vi "Wavechart erstellen.vi"(1 "file path (dialog if empty)":path) -> (0 "XY Graph":cluster{timestamp[], dbl[]}[](graph))   [LabVIEW 2021]
uses:
  <vilib>/Utility/file.llb/Read Delimited Spreadsheet (string).vi
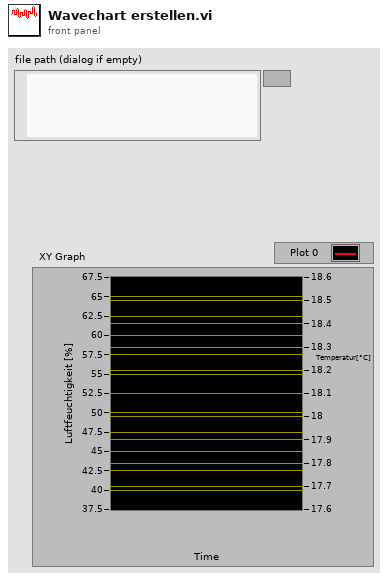
[diagram p1: front panel]
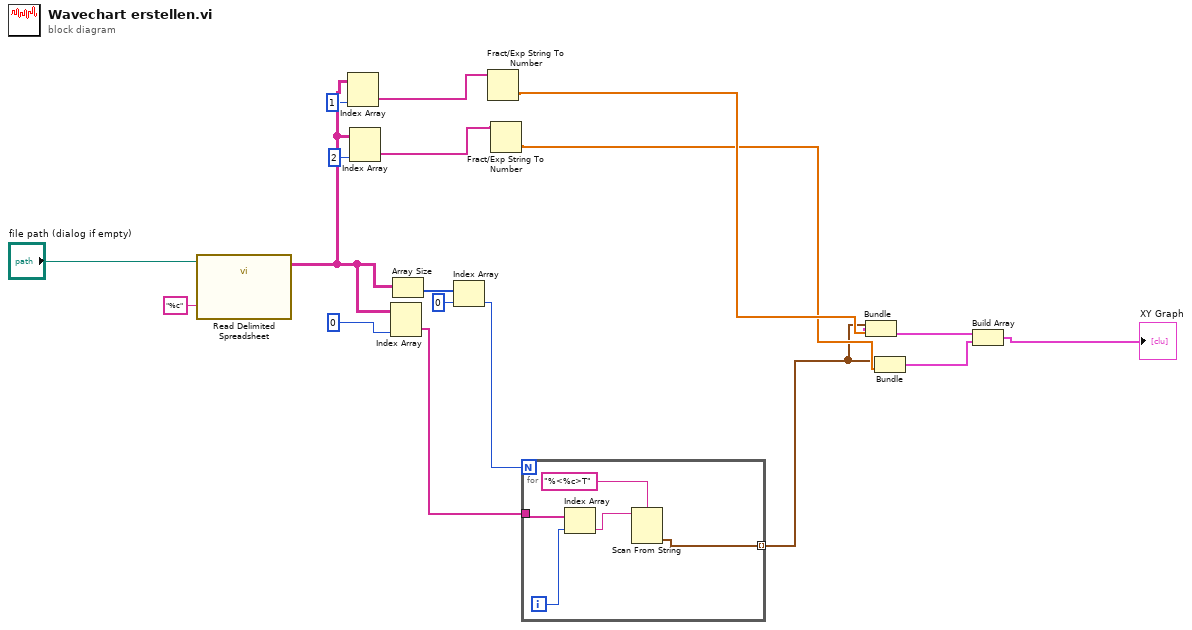
[diagram p0: block diagram]
diagram:
  n1 = call-poly <vilib>:"Read Delimited Spreadsheet.vi"("file path (dialog if empty)"="file path (dialog if empty)", "format (%s)"="%c") -> ("all rows"=w11:string[][])  [unwired: 8 in, 5 out]
  n2 = Index Array(array=w11, index (col)=1 ("disabled index (col)")) -> (element=w7:string[])  [unwired: 1 in]
  n3 = Index Array(array=w11, index (col)=2 ("disabled index (col)")) -> (element=w8:string[])  [unwired: 1 in]
  n4 = Index Array(array=w11, index (col)=0 ("index (row)")) -> (element=w13:string[])  [unwired: 1 in]
  n5 = Array Size(array=w11) -> (size(s)=w16:i32[])
  n6 = Index Array(array=w16, index=0) -> (element=w14:i32)
  n7 = Fract/Exp String To Number(string=w7) -> (number=w6:dbl[])  [unwired: 3 in, 1 out]
  n8 = Fract/Exp String To Number(string=w8) -> (number=w5:dbl[])  [unwired: 3 in, 1 out]
  n9 = for {
    N: w14 -> [_]
    tunnel: w13 -> [w21]
    tunnel: [w23] -> w4 mode=indexing
    i -> [w19]
    n10 = Index Array(array=w21, index=w19) -> (element=w20:string)
    n11 = Scan From String(format string="%<%c>T", input string=w20) -> (output 1=w23:timestamp)  [unwired: 3 in, 3 out]
  }
  n12 = Bundle(w4, w6) -> (w3:cluster{timestamp[], dbl[]})  [unwired: 1 in]
  n13 = Bundle(w4, w5) -> (w2:cluster{timestamp[], dbl[]})  [unwired: 1 in]
  n14 = Build Array(w3, w2) -> (→"XY Graph":cluster{timestamp[], dbl[]}[])
